vi "Meas Result Add Readings To Data.vi"(1 "fid (column)":i32=1, 2 "new element":T1[](array[typedef]), 3 "data in":T1[][](array[typedef])) -> (0 "data out":T1[][](array[typedef]))   [LabVIEW 2013]
doc: "Insert one reading per phase to results array with auto expansion of the array acording the data."
uses:
  bridge/Bridge Frequency Readings Data.ctl
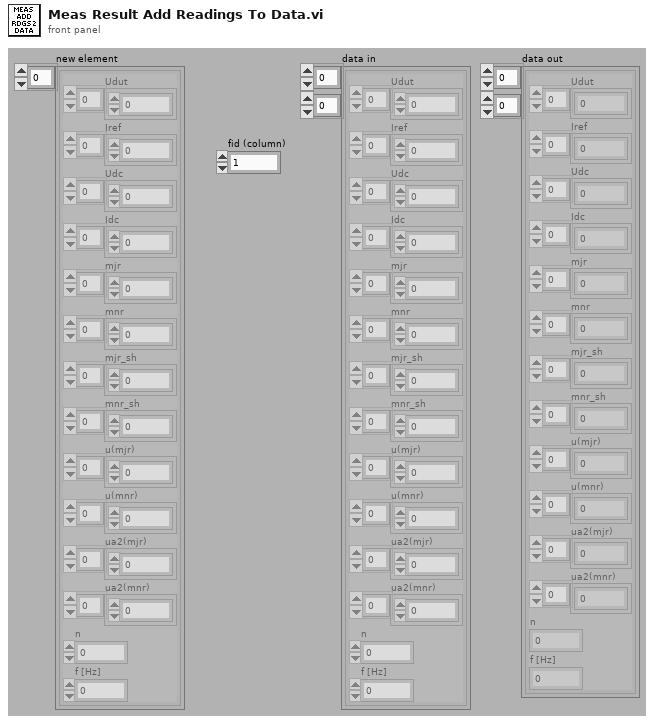
[diagram p1: front panel]
types:
  T1 = typedef "Bridge Frequency Readings Data.ctl" = cluster{"Udut":dbl[], "Iref":dbl[], "Udc":dbl[], "Idc":dbl[], "mjr":dbl[], "mnr":dbl[], "mjr_sh":dbl[], "mnr_sh":dbl[], "u(mjr)":dbl[], "u(mnr)":dbl[], "ua2(mjr)":dbl[], "ua2(mnr)":dbl[], "n":i32, "f [Hz]":dbl}
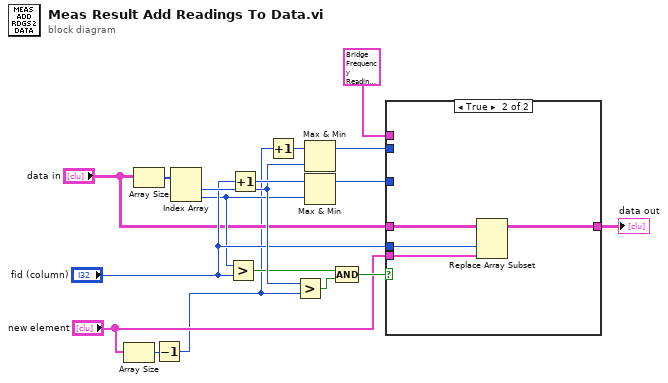
[diagram p0: block diagram]
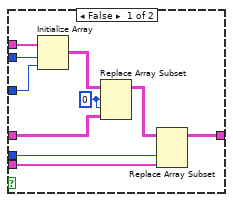
[diagram p2: hidden frame]
diagram:
  n1 = Array Size(array="new element") -> (size(s)=w2:i32)
  n2 = Array Size(array="data in") -> (size(s)=w7:i32[])
  n3 = Decrement(x=w2) -> (x-1=w1:i32)
  n4 = Index Array(array=w7) -> (element #1=w13:i32, element #2=w11:i32)  [unwired: 2 in]
  n5 = Greater?(x=w11, y="fid (column)") -> (0:w8:bool)
  n6 = Increment(x="fid (column)") -> (x+1=w16:i32)
  n7 = Increment(x=w1) -> (x+1=w17:i32)
  n8 = Greater?(x=w13, y=w1) -> (0:w9:bool)
  n9 = Max & Min(x=w17, y=w13) -> (max(x,y)=w14:i32)  [unwired: 1 out]
  n10 = Max & Min(x=w16, y=w11) -> (max(x,y)=w15:i32)  [unwired: 1 out]
  n11 = Compound Arithmetic op=AND(w8, w9) -> (w10:bool)
  n12 = case shown="True" w10 {
    tunnel: "data in" -> [w20 w31]
    tunnel: "new element" -> [w27 w29]
    tunnel: [w26 w30] -> w4
    tunnel: "fid (column)" -> [w25 w28]
    tunnel: w14 -> [w24 _]
    tunnel: w15 -> [w23 _]
    tunnel: T1 {"Udut"=[], "Iref"=[], "Udc"=[], "Idc"=[], "mjr"=[], "mnr"=[], "mjr_sh"=[], "mnr_sh"=[], "u(mjr)"=[], "u(mnr)"=[], "ua2(mjr)"=[], "ua2(mnr)"=[], "n"=0, "f [Hz]"=0.0} ("element") -> [w22 _]
    frame False {
      w19 = 0 ("index (row)")
      n13 = Initialize Array(w22, w24, w23) -> (w21:T1[][])
      n14 = Replace Array Subset(array=w21, new element=w20, index (row)=w19, index (col)=w19) -> (w18:T1[][])
      n15 = Replace Array Subset(array=w18, new element=w27, index (col)=w25) -> (w26:T1[][])  [unwired: 1 in]
    }
    frame True {
      n16 = Replace Array Subset(array=w31, new element=w29, index (col)=w28) -> (w30:T1[][])  [unwired: 1 in]
    }
  }
  "data out" <- w4
